vi "ziExample1-Module-MDS.vi"() -> ()   [LabVIEW 2016]
doc: "This examples allows to control a Zurich Instruments device via a LabOne Labview API. \nThis vi enables the multi-device synchronisation of two ZI instruments of the same family.\n\n© Zurich Instruments AG, www.zhinst.com"
uses:
  <instrlib>/Zurich Instruments LabOne/Public/Modules/ziTypeModEnum.ctl
  <instrlib>/Zurich Instruments LabOne/Public/Modules/ziModSetValueDouble.vi
  <instrlib>/Zurich Instruments LabOne/Public/Modules/ziModSetValueBinary.vi
  <instrlib>/Zurich Instruments LabOne/Public/Modules/ziModGetNodeValueString.vi
  <instrlib>/Zurich Instruments LabOne/Public/Modules/ziModGetNodeValueDouble.vi
  <instrlib>/Zurich Instruments LabOne/Zurich Instruments LabOne.lvlib
panel:
  in  "Slaves":string[](array[string])=["dev"]
  out "Status":dbl
  out "Message":string
  in  "Master":string="dev"
  # "ziExample-Module-MDS.vi\nRequirements: 2xHF2\nsee block diagram for VI description"
  # "Tested Devices:\n\n- HF2\n- MFLI\n- UHF"
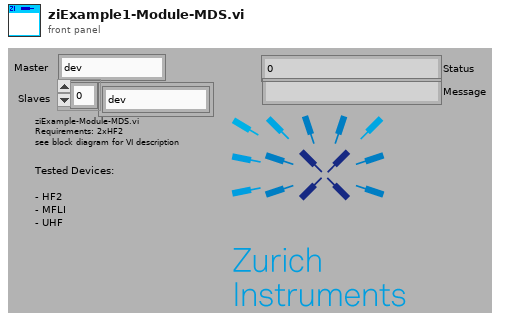
[diagram p1: front panel]
types:
  T1 = typedef "Zurich Instruments LabOne.lvlib/ziTypeModEnum.ctl" = u16
  T2 = typedef "Zurich Instruments LabOne.lvlib/ziTypeHandle.ctl" = cluster{"handleValid":bool, "Conn":u64, "Path Prefix":string, "Handle":u64, "Connected":bool, "Clockbase(s)":dbl}
  T3 = typedef "ziTypeDisovery.ctl" = cluster{"timestamp":u64, "deviceid":string, "devicetype":string, "serveraddress":string, "serverport":u32, "apilevel":u32, "discoverable":bool, "interface":string, "connected":string, "available":bool, "owner":string, "status":string, "options ":string, "serverversion":string}
  T4 = typedef "Zurich Instruments LabOne.lvlib/ziTypeModHandle.ctl" = cluster{"handleValid":bool, "Conn":u64, "ModHandle":u64, "moduleID":string, "Path Prefix":string}
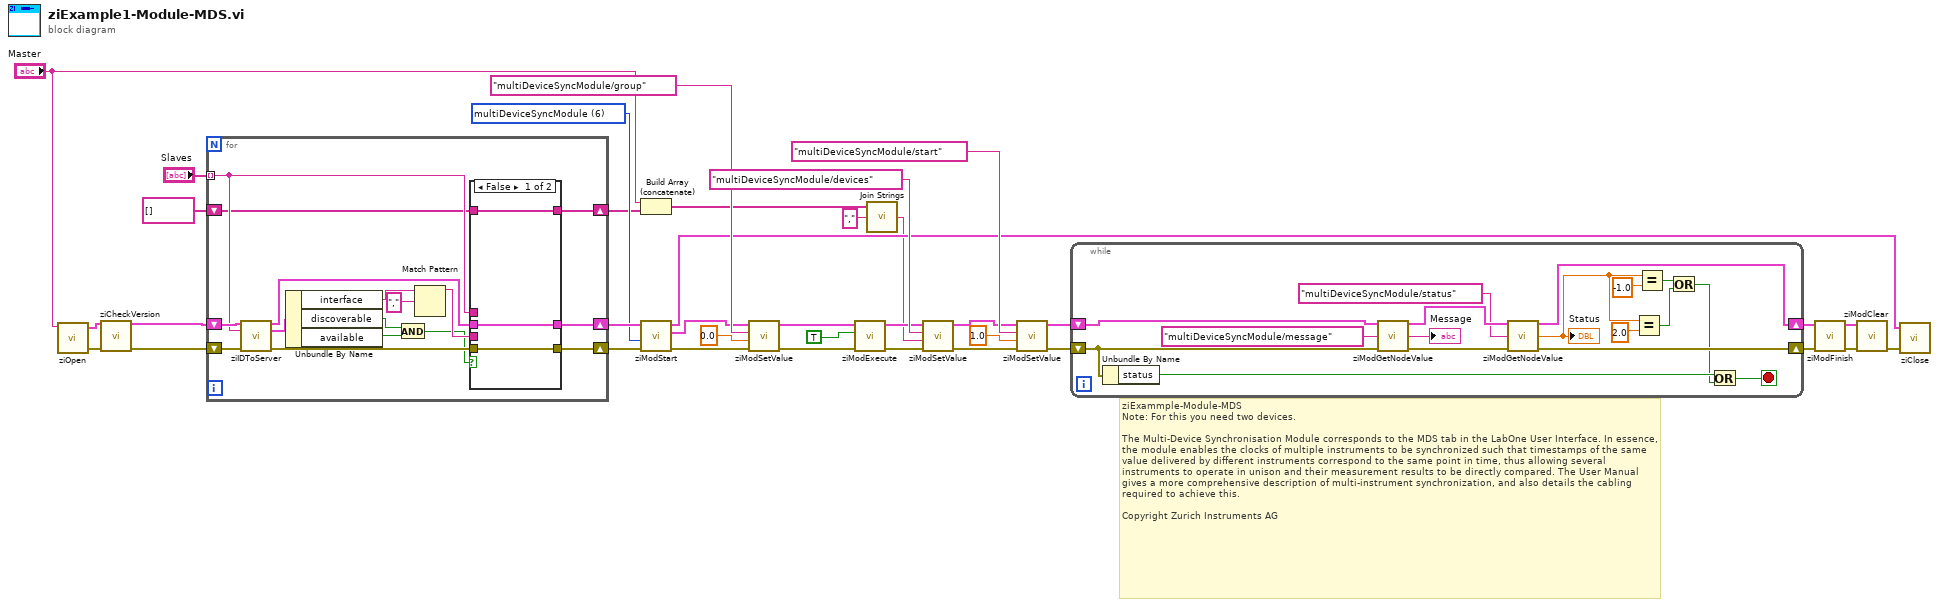
[diagram p0: block diagram]
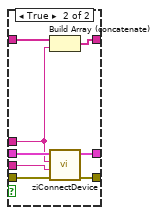
[diagram p2: hidden frame]
diagram:
  w5 = T1 6 items=["sweep", "scopeModule", "dataAcquisitionModule", "pidAdvisor", "awgModule", "impedanceModule", "multiDeviceSyncModule", "zoomFFT", "trigger", "deviceSettings", "record"] ("module Id")
  # "ziExammple-Module-MDS\nNote: For this you need two devices.\n \nThe Multi-Device Synchronisation Module corresponds to the MDS tab in the LabOne User Interface. In essence, the module enables the clocks of multiple instruments to be synchronized such that timestamps of the same value delivered by different instruments correspond to the same point in time, thus allowing several instruments to operate in unison and their measurement results to be directly compared. The User Manual gives a more comprehensive description of multi-instrument synchronization, and also details the cabling required to achieve this.\n\nCopyright Zurich Instruments AG"
  n1 = call <instrlib>:"ziOpen.vi"("Address"="Master") -> ("Error Out"=w11:errorcluster, "HandleOut"=w12:T2)  [unwired: 3 in, 1 out]
  n2 = call <instrlib>:"ziCheckVersion.vi"("Handle In"=w12, "Error In"=w11) -> ("Handle Out"=w10:T2, "Error Out"=w9:errorcluster)  [unwired: 11 in, 1 out]
  n3 = for {
    shift-right: [w52] -> w36
    shift-left: w10 -> [w50]
    shift-right: [w51] -> w35
    shift-left: w9 -> [w49]
    tunnel: "Slaves" -> [w42] mode=indexing
    shift-right: [w38] -> w2
    shift-left: string[] [] -> [w37]
    n4 = call <instrlib>:"ziIDToServer.vi"("ziHandle In"=w50, "Device ID"=w42, "Error In"=w49) -> ("ziHandle Out"=w48:T2, "ziDiscovery"=w46:T3, "Error Out"=w47:errorcluster)  [unwired: 10 in]
    n5 = Unbundle By Name(w46) -> ("interface"=w45:string, "discoverable"=w41:bool, "available"=w40:bool)
    n6 = And(x=w41, y=w40) -> (x .and. y?=w39:bool)
    n7 = Match Pattern(string=w45, regular expression=",") -> (before substring=w43:string)  [unwired: 1 in, 3 out]
    n8 = case shown="False" w39 {
      tunnel: [w55 w63] -> w52
      tunnel: [w54 w62] -> w51
      tunnel: w48 -> [w55 w61]
      tunnel: w47 -> [w54 w60]
      tunnel: w43 -> [_ w59]
      tunnel: w42 -> [_ w56]
      tunnel: [w53 w58] -> w38
      tunnel: w37 -> [w53 w57]
      frame False {
      }
      frame True {
        n9 = Build Array (concatenate)(w57, w56) -> (w58:string[])
        n10 = call <instrlib>:"ziConnectDevice.vi"("Error In"=w60, "Device Interface"=w59, "Device Serial"=w56, "Handle In"=w61) -> ("Error Out"=w62:errorcluster, "Handle Out"=w63:T2)  [unwired: 6 in]
      }
    }
  }
  n11 = Build Array (concatenate)("Master", w2) -> (w1:string[])
  n12 = call <instrlib>:"ziModStart.vi"("Error In"=w35, "module Id"=w5, "Handle In"=w36) -> ("Error Out"=w26:errorcluster, "ModHandle Out"=w23:T4, "Handle Out"=w15:T2)  [unwired: 6 in]
  n13 = call-poly <instrlib>:"ziModSetValue.vi"("Error In"=w26, "Value"=0.0, "Path"="multiDeviceSyncModule/group", "ModHandle In"=w23) -> ("Error Out"=w25:errorcluster, "ModHandle Out"=w22:T4)  [unwired: 6 in]
  n14 = call <instrlib>:"ziModExecute.vi"("Error In"=w25, "Modal (F)"=TRUE, "ziModHandle In"=w22) -> ("Error Out"=w24:errorcluster, "ziModHandle Out"=w21:T4)  [unwired: 5 in, 1 out]
  n15 = call <vilib>:"Join Strings.vi"("Separator (,)"="," ("string"), "Strings In"=w1) -> ("String"=w6:string)  [unwired: 1 in]
  n16 = call-poly <instrlib>:"ziModSetValue.vi"("Error In"=w24, "Data"=w6, "Path"="multiDeviceSyncModule/devices", "ModHandle In"=w21) -> ("Error Out"=w30:errorcluster, "ModHandle Out"=w31:T4)  [unwired: 6 in]
  n17 = call-poly <instrlib>:"ziModSetValue.vi"("Error In"=w30, "Value"=1.0, "Path"="multiDeviceSyncModule/start", "ModHandle In"=w31) -> ("Error Out"=w19:errorcluster, "ModHandle Out"=w20:T4)  [unwired: 6 in]
  n18 = while {
    shift-right: [w72] -> w13
    shift-left: w20 -> [w79]
    shift-right: [w73] -> w18
    shift-left: w19 -> [w66]
    stop <- w64 stop-if-true
    n19 = Unbundle By Name(w66) -> ("status"=w67:bool)
    n20 = call-poly <instrlib>:"ziModGetNodeValue.vi"("ModHandle In"=w79, "Path"="multiDeviceSyncModule/message", "error in"=w66) -> ("ModHandle Out"=w78:T4, "Value"=→"Message":string, "error out"=w77:errorcluster)  [unwired: 10 in]
    n21 = call-poly <instrlib>:"ziModGetNodeValue.vi"("ModHandle In"=w78, "Path"="multiDeviceSyncModule/status", "error in"=w77) -> ("ModHandle Out"=w72:T4, "Value"=w69:dbl, "error out"=w73:errorcluster)  [unwired: 10 in]
    "Status" <- w69
    n22 = Equal?(x=w69, y=2.0) -> (x = y?=w70:bool)
    n23 = Equal?(x=w69, y=-1.0) -> (x = y?=w71:bool)
    n24 = Or(x=w71, y=w70) -> (x .or. y?=w65:bool)
    n25 = Or(x=w67, y=w65) -> (x .or. y?=w64:bool)
  }
  n26 = call <instrlib>:"ziModFinish.vi"("Error In"=w18, "ziModHandle In"=w13) -> ("Error Out"=w17:errorcluster, "ziModHandle Out"=w14:T4)  [unwired: 7 in]
  n27 = call <instrlib>:"ziModClear.vi"("Error In"=w17, "ziModHandle In"=w14) -> ("Error Out"=w16:errorcluster)  [unwired: 7 in, 1 out]
  n28 = call <instrlib>:"ziClose.vi"("Error In"=w16, "Handle In"=w15) -> ()  [unwired: 2 in, 2 out]
